vi "divider_and_offset_Rev_03.vi"(0 "Char Array In":dbl[](array[numeric]), 5 "Control Char":string) -> (1 "Div In2 Rgt Ind":dbl format="%.2f", 3 "Div In1 Lft Ind":dbl format="%.2f", 4 "Div In1 Lft":dbl, 6 "Div In2 Rgt":dbl, 9 "INPUT2 shift sign":dbl, 10 "Shft IN1 L uV":dbl format="%#_6f", 11 "INPUT1 shift sign":dbl, 12 "Shift IN2 R ch1":dbl format="%#_6f", 14 "Shift IN1 L ch0":dbl)   [LabVIEW 2012]
panel:
  out "Number of cal bytes":dbl
  # "CH0 LB"
  # "CH0 HB"
  # "CH0 UB"
  # "CH0 MB"
  # "CH0 sign"
  # "CH1 LB"
  # "CH1 HB"
  # "CH1 UB"
  # "CH1 MB"
  # "CH1 sign"
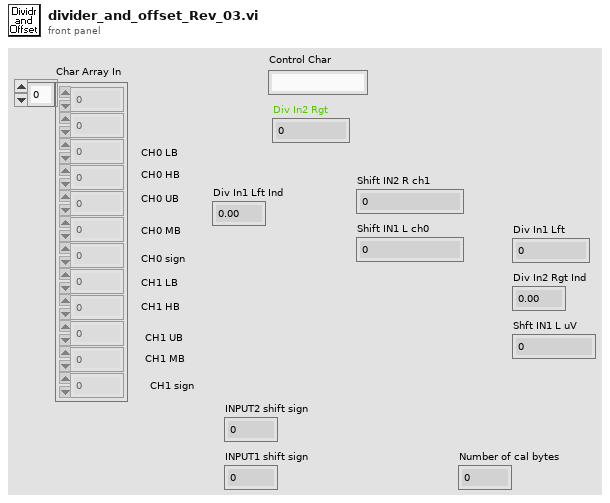
[diagram p1: front panel]
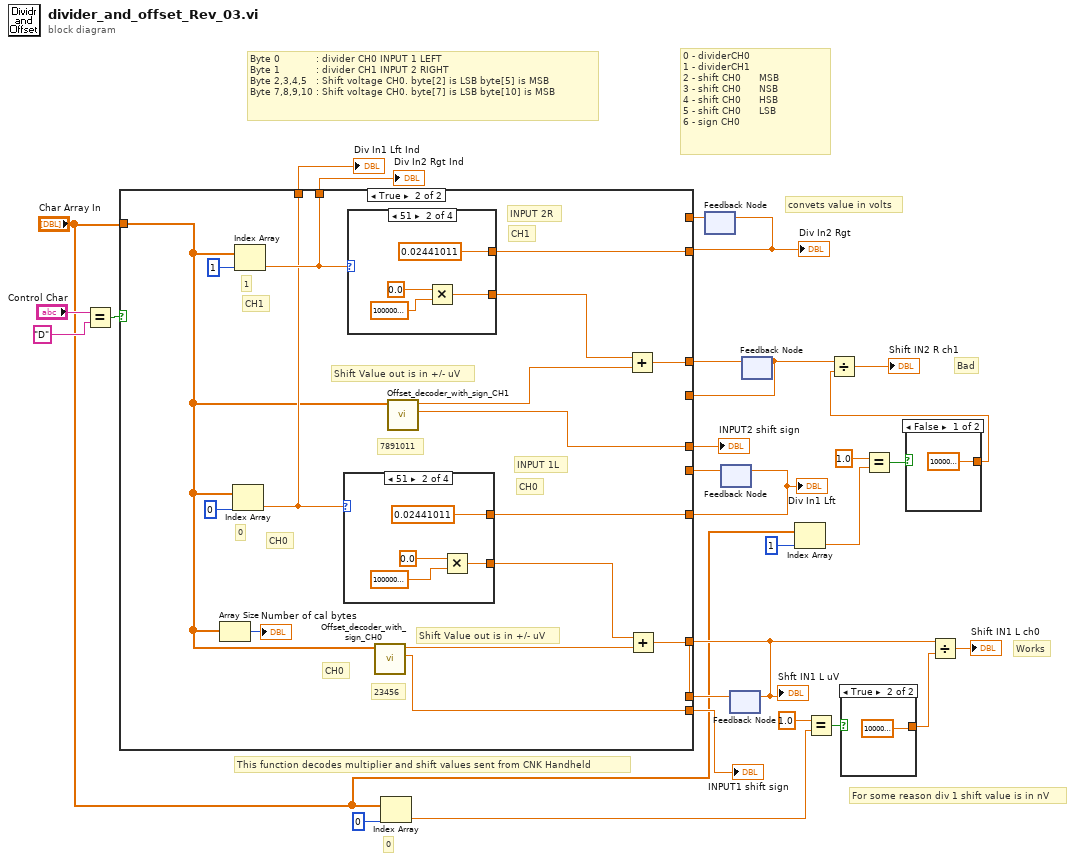
[diagram p0: block diagram]
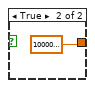
[diagram p2: hidden frame]
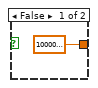
[diagram p3: hidden frame]
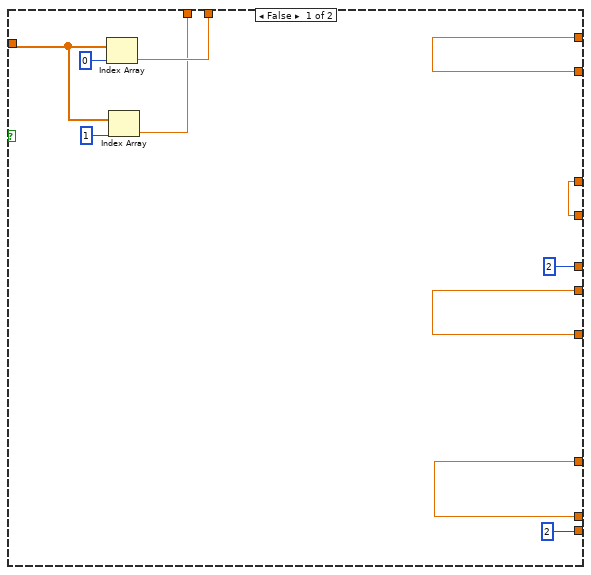
[diagram p4: hidden frame]
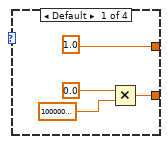
[diagram p5: hidden frame]
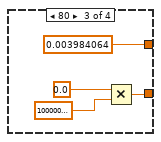
[diagram p6: hidden frame]
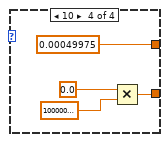
[diagram p7: hidden frame]
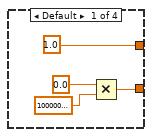
[diagram p8: hidden frame]
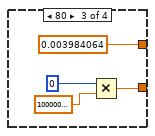
[diagram p9: hidden frame]
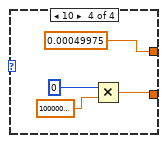
[diagram p10: hidden frame]
diagram:
  # "Bad"
  # "Works"
  # "For some reason div 1 shift value is in nV"
  # "0"
  # "Byte 0            : divider CH0 INPUT 1 LEFT\nByte 1            : divider CH1 INPUT 2 RIGHT\nByte 2,3,4,5   : Shift voltage CH0. byte[2] is LSB byte[5] is MSB\nByte 7,8,9,10 : Shift voltage CH0. byte[7] is LSB byte[10] is MSB"
  # "0 - dividerCH0   \n1 - dividerCH1\n2 - shift CH0      MSB\n3 - shift CH0      NSB\n4 - shift CH0      HSB    \n5 - shift CH0      LSB\n6 - sign CH0"
  # "This function decodes multiplier and shift values sent from CNK Handheld"
  # "convets value in volts"
  n1 = Equal?(x="Control Char", y="D") -> (x = y?=w27:bool)
  n2 = Index Array(array="Char Array In", index=0) -> (element=w9:dbl)
  n3 = feedback #1() -> (w25:dbl)  [unwired: 1 in]
  n4 = feedback #2() -> (w24:dbl)  [unwired: 1 in]
  n5 = feedback #3() -> (w22:dbl)  [unwired: 1 in]
  "Shft IN1 L uV" <- w22
  n6 = feedback #4() -> (w3:dbl)  [unwired: 1 in]
  n7 = case shown="True" w27 {
    tunnel: [w39 w53] -> w16
    tunnel: [w38 w52] -> w17
    tunnel: w25 -> [w39 _]
    tunnel: w24 -> [w38 _]
    tunnel: "Char Array In" -> [w32 w46]
    tunnel: [w37 w49] -> w23
    tunnel: w22 -> [w37 _]
    tunnel: [w29 w44] -> w4
    tunnel: [w34 w51] -> w21
    tunnel: [w33 w50] -> w20
    tunnel: [2 w48] -> w19
    tunnel: [2 w47] -> w18
    tunnel: w3 -> [w29 _]
    frame False {
      n8 = Index Array(array=w32, index=0) -> (element=w34:dbl)
      n9 = Index Array(array=w32, index=1) -> (element=w33:dbl)
    }
    frame True {
      # "CH0"
      # "CH0"
      # "CH0"
      # "CH1"
      # "CH1"
      # "1"
      # "0"
      # "7891011"
      # "23456"
      # "Shift Value out is in +/- uV"
      # "Shift Value out is in +/- uV"
      # "INPUT 1L"
      # "INPUT 2R"
      n10 = Array Size(array=w46) -> (size(s)=→"Number of cal bytes":i32)
      n11 = Index Array(array=w46, index=0) -> (element=w50:dbl)
      n12 = Index Array(array=w46, index=1) -> (element=w51:dbl)
      n13 = case shown="51" w50 {
        tunnel: [1.0 0.02441011 0.003984064 0.00049975] -> w52
        tunnel: [w56 w60 w64 w68] -> w40
        frame Default {
          n14 = Multiply(x=0.0, y=10000000000.0) -> (x*y=w56:dbl)
        }
        frame 51 {
          n15 = Multiply(x=0.0, y=10000000000.0) -> (x*y=w60:dbl)
        }
        frame 80 {
          n16 = Multiply(x=0.0, y=10000000000.0) -> (x*y=w64:dbl)
        }
        frame 10 {
          n17 = Multiply(x=0.0, y=10000000000.0) -> (x*y=w68:dbl)
        }
      }
      n18 = case shown="51" w51 {
        tunnel: [1.0 0.02441011 0.003984064 0.00049975] -> w53
        tunnel: [w72 w76 w80 w84] -> w43
        frame Default {
          n19 = Multiply(x=0.0 ("SHIFT INPUT 1L"), y=10000000000.0) -> (x*y=w72:dbl)
        }
        frame 51 {
          n20 = Multiply(x=0.0, y=10000000000.0) -> (x*y=w76:dbl)
        }
        frame 80 {
          n21 = Multiply(x=0, y=10000000000.0) -> (x*y=w80:dbl)
        }
        frame 10 {
          n22 = Multiply(x=0, y=10000000000.0) -> (x*y=w84:dbl)
        }
      }
      n23 = call "Offset_decoder_with_sign_CH0.vi"("Array In1"=w46) -> ("Sign"=w48:dbl, "CH0 uV"=w41:dbl)  [unwired: 9 in]
      n24 = call "Offset_decoder_with_sign_CH1.vi"("Array In1"=w46) -> ("Sign CH1"=w47:dbl, "CH1 SHIFT"=w42:dbl)  [unwired: 9 in]
      n25 = Add(x=w43, y=w42) -> (x+y=w44:dbl)
      n26 = Add(x=w40, y=w41) -> (x+y=w49:dbl)
    }
  }
  "Div In2 Rgt" <- w16
  "Div In1 Lft" <- w17
  "Div In1 Lft Ind" <- w20
  "Div In2 Rgt Ind" <- w21
  "INPUT2 shift sign" <- w18
  "INPUT1 shift sign" <- w19
  n27 = feedback-in #1(w16) -> ()
  n28 = feedback-in #2(w17) -> ()
  n29 = feedback-in #3(w23) -> ()
  n30 = feedback-in #4(w4) -> ()
  n31 = Index Array(array="Char Array In", index=1) -> (element=w5:dbl)
  n32 = Equal?(x=1.0, y=w9) -> (x = y?=w12:bool)
  n33 = case shown="True" w12 {
    tunnel: [1000000.0 1000000000.0] -> w13
    frame False {
    }
    frame True {
    }
  }
  n34 = Equal?(x=1.0, y=w5) -> (x = y?=w7:bool)
  n35 = case shown="False" w7 {
    tunnel: [1000000.0 1000000000.0] -> w1
    frame False {
    }
    frame True {
    }
  }
  n36 = Divide(x=w3, y=w1) -> (x/y=→"Shift IN2 R ch1":dbl)
  n37 = Divide(x=w22, y=w13) -> (x/y=→"Shift IN1 L ch0":dbl)
